vi "Jain's method RT.vi"(8 "Prev Amp":dbl, 9 "Next Amp":dbl, 10 "Max Amp":fxp<+,46,22>, 11 "Max Bin":i32) -> (2 "Bin":fxp<+/-,64,66>)   [LabVIEW 2014]
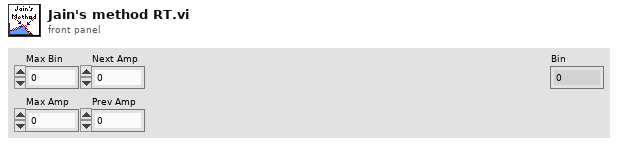
[diagram p1: front panel]
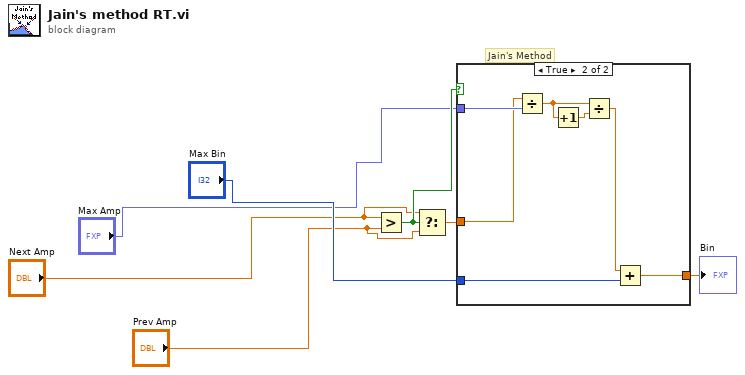
[diagram p0: block diagram]
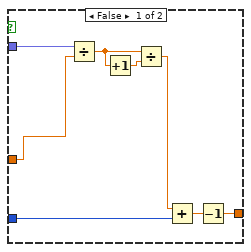
[diagram p2: hidden frame]
diagram:
  # "Jain's Method"
  n1 = Greater?(x="Next Amp", y="Prev Amp") -> (0:w7:bool)
  n2 = Select(t="Next Amp", s=w7, f="Prev Amp") -> (s? t:f=w6:dbl)
  n3 = case shown="True" w7 {
    tunnel: w6 -> [w9 w16]
    tunnel: "Max Amp" -> [w8 w22]
    tunnel: "Max Bin" -> [w10 w18]
    tunnel: [w13 w17] -> w5
    frame False {
      n4 = Divide(x=w8, y=w9) -> (x/y=w14:dbl)
      n5 = Increment(x=w14) -> (x+1=w15:dbl)
      n6 = Divide(x=w14, y=w15) -> (x/y=w11:dbl)
      n7 = Add(x=w11, y=w10) -> (x+y=w12:dbl)
      n8 = Decrement(x=w12) -> (x-1=w13:dbl)
    }
    frame True {
      n9 = Divide(x=w16, y=w22) -> (x/y=w20:dbl)
      n10 = Increment(x=w20) -> (x+1=w21:dbl)
      n11 = Divide(x=w20, y=w21) -> (x/y=w19:dbl)
      n12 = Add(x=w19, y=w18) -> (x+y=w17:dbl)
    }
  }
  "Bin" <- w5
